vi "Pos2DatByCH.vi"(1 "Draw Area Size":T1 caption="Pic Draw Area Size", 2 "PosInCurve":cluster{i16, i16}[](array[cluster])) -> (0 "FalseColorRatioData":cluster{dbl, dbl}[](array[cluster]))   [LabVIEW 2016]
uses:
  <vilib>/Utility/miscctls.llb/LVBoundsTypeDef.ctl
panel:
  # "本VI把RGB三条伪彩色编辑曲线的节点X坐标(相对)转化为灰度级比率0~1,把Y轴坐标转化为0~255的灰度值"
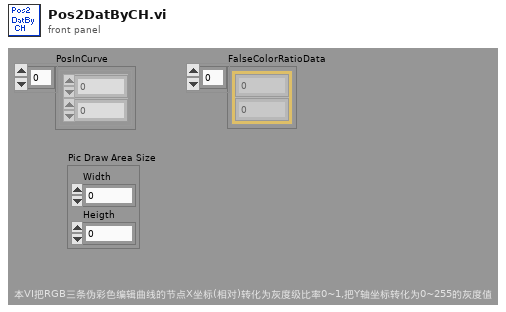
[diagram p1: front panel]
types:
  T1 = typedef "LVBoundsTypeDef.ctl" = cluster{"Width":u32, "Height":u32}
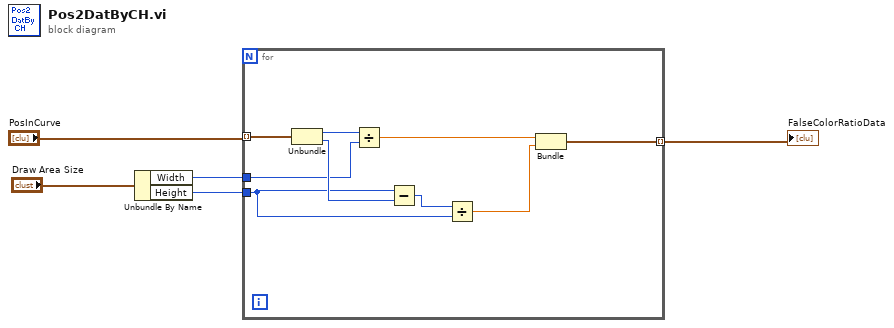
[diagram p0: block diagram]
diagram:
  n1 = Unbundle By Name("Draw Area Size") -> ("Width"=w3:u32, "Height"=w4:u32)
  n2 = for {
    tunnel: "PosInCurve" -> [w14] mode=indexing
    tunnel: [w11] -> w5 mode=indexing
    tunnel: w4 -> [w7]
    tunnel: w3 -> [w10]
    n3 = Unbundle(w14) -> (w9:i16, w12:i16)
    n4 = Divide(x=w9, y=w10) -> (x/y=w8:dbl)
    n5 = Subtract(x=w7, y=w12) -> (x-y=w13:u32)
    n6 = Divide(x=w13, y=w7) -> (x/y=w6:dbl)
    n7 = Bundle(w8, w6) -> (w11:cluster{dbl, dbl})  [unwired: 1 out]
  }
  "FalseColorRatioData" <- w5
